vi "Stop Event.vi"(7 "Actions":T1(ring)=enum."Generate Event", 8 "error in":errorcluster, 10 "Data":variant) -> (0 "error out":errorcluster, 3 "Stop":refnum<user-event>)   [LabVIEW 2020]
doc: "Stop user event FGV.\n\n-----\nJuan Navarro\nLab it Studio"
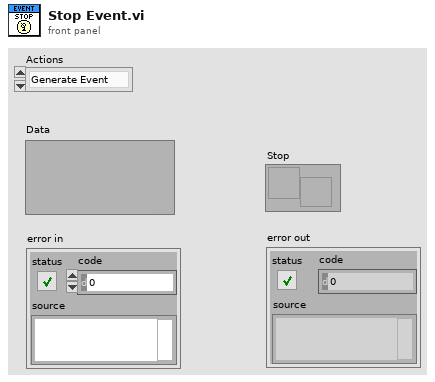
[diagram p1: front panel]
types:
  T1 = enum16{"Create Event", "Generate Event", "Destroy Event"}
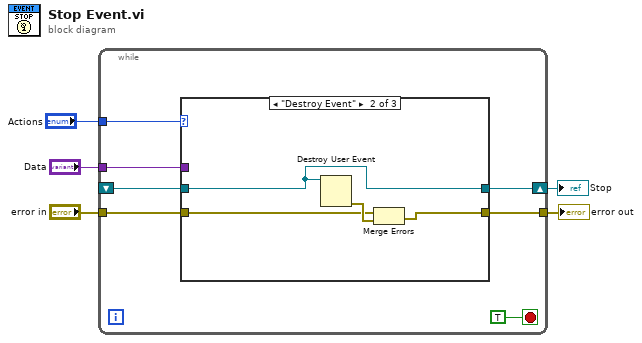
[diagram p0: block diagram]
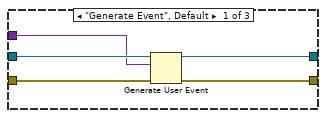
[diagram p2: hidden frame]
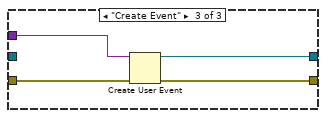
[diagram p3: hidden frame]
diagram:
  n1 = while {
    tunnel: "Data" -> [w12]
    tunnel: "error in" -> [w11]
    tunnel: [w10] -> w4
    shift-right: [w9] -> w2
    shift-left: _ -> [w8]
    tunnel: "Actions" -> [w6]
    stop <- TRUE stop-if-true
    n2 = case shown="\"Destroy Event\"" w6 {
      tunnel: w12 -> [w13 _ w25]
      tunnel: w11 -> [w17 w18 w24]
      tunnel: [w16 w20 w23] -> w10
      tunnel: [w14 w21 w22] -> w9
      tunnel: w8 -> [w15 w21 _]
      frame "Generate Event", Default {
        n3 = Generate User Event(user event=w15, event data cluster=w13, error in=w17) -> (user event out=w14:refnum<user-event>, error out=w16:errorcluster)  [unwired: 1 in]
      }
      frame "Destroy Event" {
        n4 = Destroy User Event(user event=w21) -> (error out=w19:errorcluster)  [unwired: 1 in]
        n5 = Merge Errors(w18, w19) -> (w20:errorcluster)
      }
      frame "Create Event" {
        n6 = Create User Event(user event datatype=w25, error in=w24) -> (user event=w22:refnum<user-event>, error out=w23:errorcluster)
      }
    }
  }
  "error out" <- w4
  "Stop" <- w2
